vi "CleanIT (SubVI).vi"(1 "in array":dbl[][](array[numeric])) -> (0 "pre-cleaned Array":dbl[][](array[numeric]))   [LabVIEW 2011]
uses:
  <vilib>/Analysis/NI_AALBase.lvlib
panel:
  out "size w/o zeroes":i32[](array[numeric])
  out "ori size":i32[](array[numeric])
  out "final size":i32[](array[numeric])
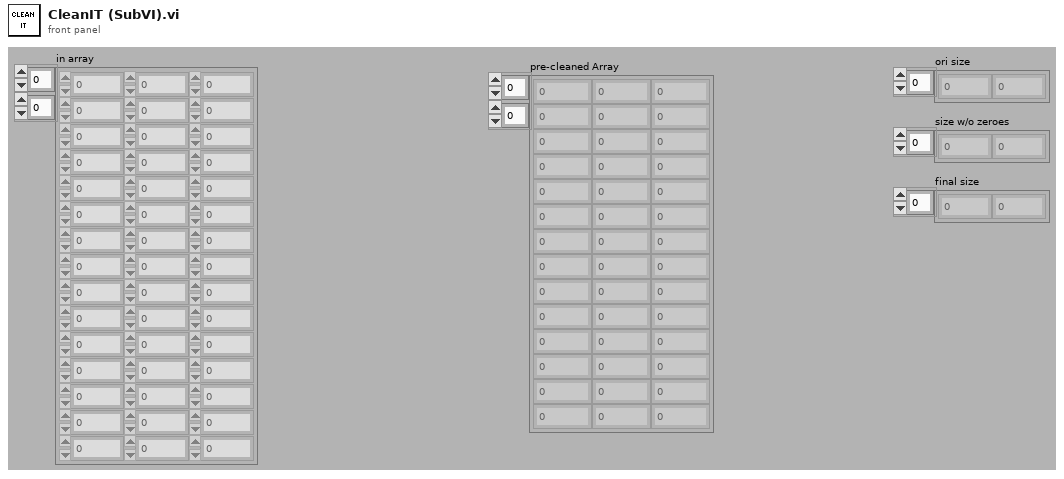
[diagram p1: front panel]
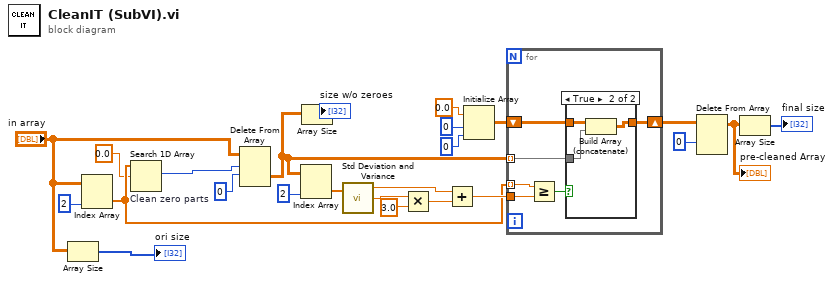
[diagram p0: block diagram]
diagram:
  n1 = Array Size(array="in array") -> (size(s)=→"ori size":i32[])
  n2 = Index Array(array="in array", index (col)=2 ("disabled index (col)")) -> (element=w9:dbl[])  [unwired: 1 in]
  n3 = Search 1D Array "Clean zero parts"(1D array=w9, element=0.0) -> (index of element=w3:i32)  [unwired: 1 in]
  n4 = Delete From Array(array="in array", length=w3, index (row)=0) -> (deleted portion=w1:dbl[][])  [unwired: 1 in, 1 out]
  n5 = Index Array(array=w1, index (col)=2 ("disabled index (col)")) -> (element=w5:dbl[])  [unwired: 1 in]
  n6 = Array Size(array=w1) -> (size(s)=→"size w/o zeroes":i32[])
  n7 = call <vilib>:"Std Deviation and Variance.vi"("X"=w5) -> ("mean"=w23:dbl, "standard deviation"=w22:dbl)  [unwired: 1 in, 1 out]
  n8 = Multiply(x=w22, y=3.0) -> (x*y=w20:dbl)
  n9 = Add(x=w23, y=w20) -> (x+y=w19:dbl)
  n10 = Initialize Array(0.0 ("element"), 0 ("dimension size"), 0 ("dimension size")) -> (w18:dbl[][])
  n11 = for {
    tunnel: w1 -> [w26] mode=indexing
    tunnel: w9 -> [w30] mode=indexing
    tunnel: w19 -> [w29]
    shift-right: [w27] -> w14
    shift-left: w18 -> [w28]
    n12 = Greater Or Equal?(x=w30, y=w29) -> (x >= y?=w25:bool)
    n13 = case shown="True" w25 {
      tunnel: w28 -> [w31 w34]
      tunnel: [w31 w33] -> w27
      tunnel: w26 -> [_ w32]
      frame False {
      }
      frame True {
        n14 = Build Array (concatenate)(w34, w32) -> (w33:dbl[][])
      }
    }
  }
  n15 = Delete From Array(array=w14, index (row)=0) -> (array with subset deleted=w12:dbl[][])  [unwired: 2 in, 1 out]
  "pre-cleaned Array" <- w12
  n16 = Array Size(array=w12) -> (size(s)=→"final size":i32[])
